vi "Write DeviceName.vi"(8 "error in (no error)":errorcluster, 10 "DeviceName":string, 11 "CCD in":refnum<class "CCD.lvclass">) -> (0 "error out":errorcluster, 3 "CCD out":refnum<class "CCD.lvclass">)   [LabVIEW 2023, in "CCD.lvclass"]
uses:
  CCD.lvclass
  GenericDevice/GenericDevice.lvclass
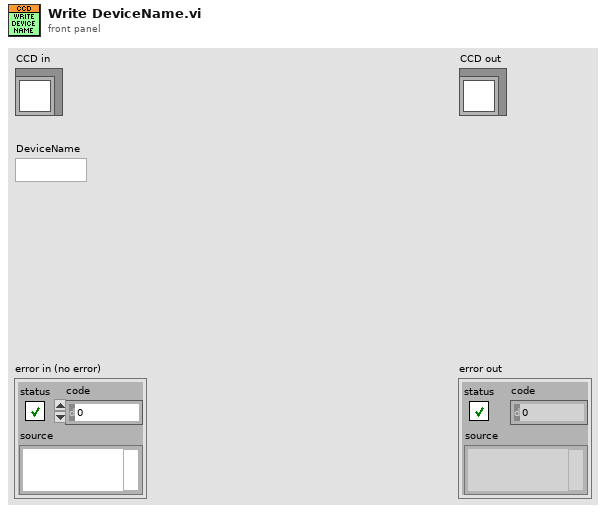
[diagram p1: front panel]
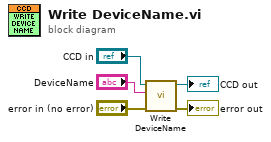
[diagram p0: block diagram]
diagram:
  n1 = call-parent "Write DeviceName.vi"("error in (no error)"="error in (no error)", "DeviceName"="DeviceName", "GenericDevice in"="CCD in") -> ("error out"=→"error out":errorcluster, "GenericDevice out"=→"CCD out":refnum<class "CCD.lvclass">)  [unwired: 7 in]
